vi "from string.vi"(8 "error in":errorcluster, 9 "data":string, 10 "version":string, 11 "configuration in":refnum<class "RIO Target Configuration.lvclass">) -> (0 "error out":errorcluster, 3 "configuration out":refnum<class "RIO Target Configuration.lvclass">)   [LabVIEW 2014, in "RIO Target Configuration.lvclass"]
doc: "Provides an interface for loading a module configuration from a file or other serialized data source. It is recommended that all children of this class store data in two sets--data required for its own initialization, and any data required for parent initialization--and that each implementation uses the <b>Call Parent Method</b> primitive to de-serialize parent information."
uses:
  RIO Target Configuration.lvclass
  RIO Target Configuration.lvclass/RIO Target Configuration.ctl
  <vilib>/NI/Configuration Framework/serializable configuration/NISE_CEF_serializable configuration.lvclass
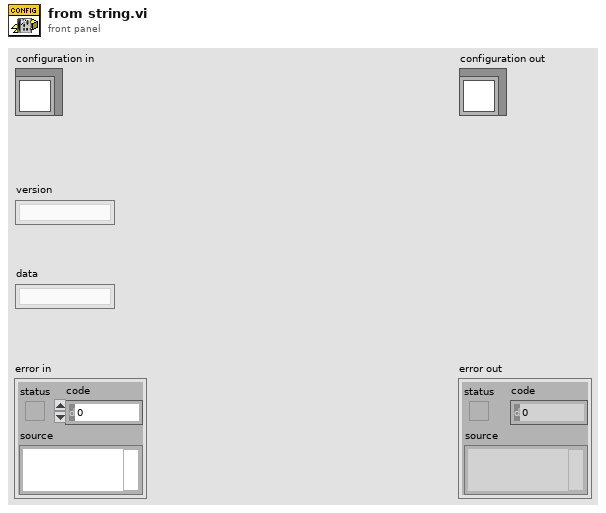
[diagram p1: front panel]
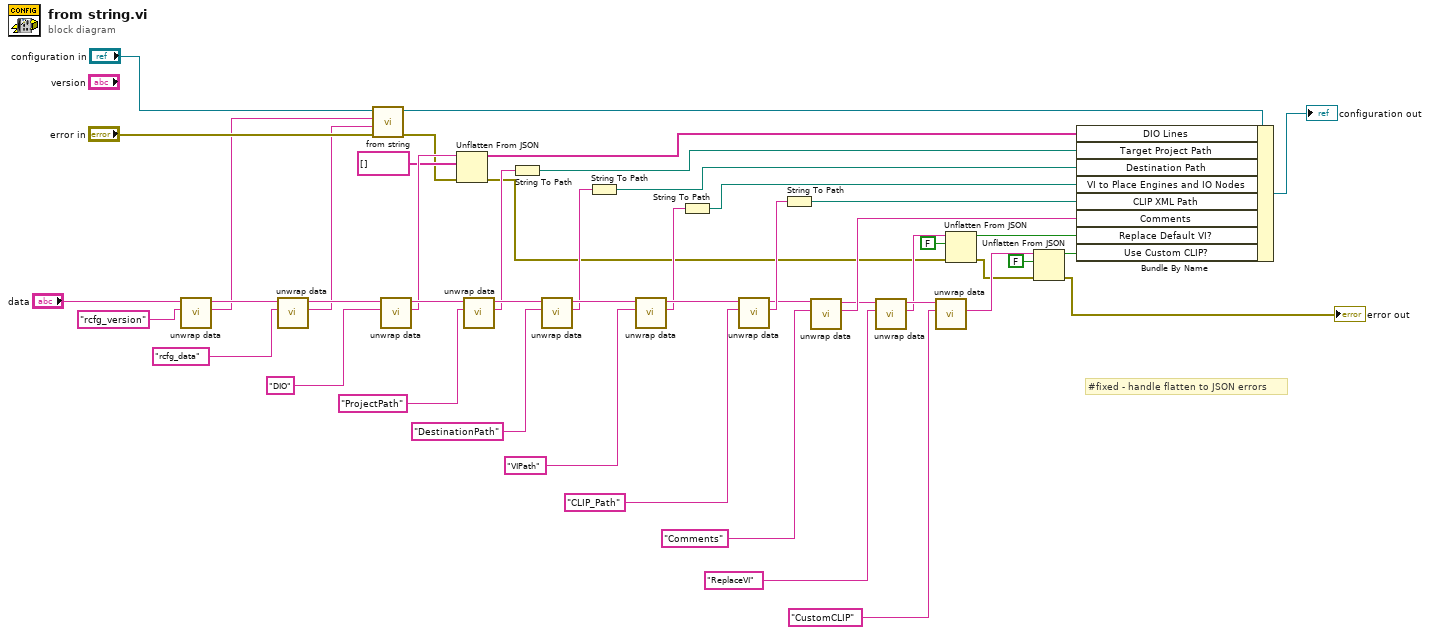
[diagram p0: block diagram]
diagram:
  # "#fixed - handle flatten to JSON errors"
  n1 = call <vilib>:"unwrap data.vi"("identifier"="rcfg_version" ("additional identifier"), "data to unwrap"="data") -> ("unwrapped data"=w32:string, "remaining string"=w45:string)  [unwired: 8 in]
  n2 = call <vilib>:"unwrap data.vi"("identifier"="rcfg_data" ("additional identifier"), "data to unwrap"=w45) -> ("unwrapped data"=w31:string, "remaining string"=w42:string)  [unwired: 8 in]
  n3 = call-parent "from string.vi"("error in"="error in", "data"=w31, "version"=w32, "configuration in"="configuration in") -> ("error out"=w4:errorcluster, "configuration out"=w33:refnum<class "RIO Target Configuration.lvclass">)  [unwired: 6 in]
  n4 = call <vilib>:"unwrap data.vi"("identifier"="DIO" ("key"), "data to unwrap"=w42) -> ("unwrapped data"=w30:string, "remaining string"=w40:string)  [unwired: 8 in]
  n5 = Unflatten From JSON(JSON string=w30, type and defaults=string[] [] ("DIO Lines"), error in (no error)=w4) -> (value=w28:string[], error out=w3:errorcluster)  [unwired: 4 in]
  n6 = call <vilib>:"unwrap data.vi"("identifier"="ProjectPath" ("key"), "data to unwrap"=w40) -> ("unwrapped data"=w27:string, "remaining string"=w38:string)  [unwired: 8 in]
  n7 = String To Path(string=w27) -> (path=w26:path)
  n8 = call <vilib>:"unwrap data.vi"("identifier"="DestinationPath" ("key"), "data to unwrap"=w38) -> ("unwrapped data"=w25:string, "remaining string"=w36:string)  [unwired: 8 in]
  n9 = String To Path(string=w25) -> (path=w24:path)
  n10 = call <vilib>:"unwrap data.vi"("identifier"="VIPath" ("key"), "data to unwrap"=w36) -> ("unwrapped data"=w22:string, "remaining string"=w23:string)  [unwired: 8 in]
  n11 = String To Path(string=w22) -> (path=w21:path)
  n12 = call <vilib>:"unwrap data.vi"("identifier"="CLIP_Path" ("key"), "data to unwrap"=w23) -> ("unwrapped data"=w20:string, "remaining string"=w17:string)  [unwired: 8 in]
  n13 = String To Path(string=w20) -> (path=w19:path)
  n14 = call <vilib>:"unwrap data.vi"("identifier"="Comments", "data to unwrap"=w17) -> ("unwrapped data"=w15:string, "remaining string"=w14:string)  [unwired: 8 in]
  n15 = call <vilib>:"unwrap data.vi"("identifier"="ReplaceVI", "data to unwrap"=w14) -> ("unwrapped data"=w10:string, "remaining string"=w12:string)  [unwired: 8 in]
  n16 = call <vilib>:"unwrap data.vi"("identifier"="CustomCLIP", "data to unwrap"=w12) -> ("unwrapped data"=w6:string)  [unwired: 8 in, 1 out]
  n17 = Unflatten From JSON(JSON string=w10, type and defaults=FALSE, error in (no error)=w3) -> (value=w9:bool, error out=w2:errorcluster)  [unwired: 4 in]
  n18 = Unflatten From JSON(JSON string=w6, type and defaults=FALSE, error in (no error)=w2) -> (value=w7:bool, error out=→"error out":errorcluster)  [unwired: 4 in]
  n19 = Bundle By Name(cluster=w33, "DIO Lines"=w28, "Target Project Path"=w26, "Destination Path"=w24, "VI to Place Engines and IO Nodes"=w21, "CLIP XML Path"=w19, "Comments"=w15, "Replace Default VI?"=w9, "Use Custom CLIP?"=w7) -> (→"configuration out":refnum<class "RIO Target Configuration.lvclass">)
